vi "Cast Command from Transfer Group.vi"(8 "error in (no error)":errorcluster, 9 "Transfer Group iteration":u64, 10 "Transfer Group id":i32, 11 "Plugin Thread in":refnum<class "Plugin Thread.lvclass">) -> (0 "error out":errorcluster, 2 "command parameters":T1, 3 "Plugin Thread out":refnum<class "Plugin Thread.lvclass">)   [LabVIEW 2021, in "DSF Core.lvlib" / "Plugin Thread.lvclass"]
uses:
  Thread/Plugin/Plugin Thread.lvclass
  Interface/Plugin/Command Parameters.ctl
  Interface/Plugin/Plugin Interface.lvclass
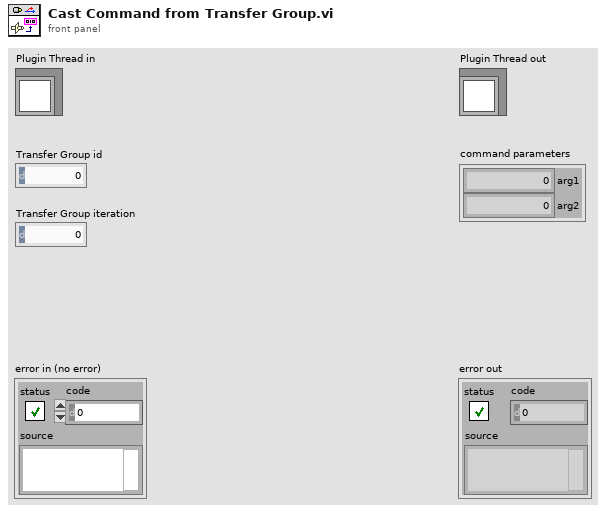
[diagram p1: front panel]
types:
  T1 = typedef "DSF Core.lvlib/Plugin Interface.lvclass/Command Parameters.ctl" = cluster{"arg1":u64, "arg2":u64}
  T2 = cluster{"Transfer Group ID":i32, "unused":i32, "Transfer Group iteration":u64}
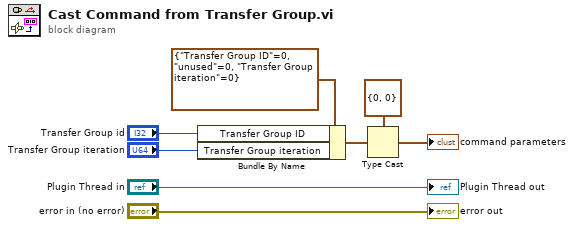
[diagram p0: block diagram]
diagram:
  n1 = Bundle By Name(cluster=T2 {"Transfer Group ID"=0, "unused"=0, "Transfer Group iteration"=0} ("Cluster"), "Transfer Group ID"="Transfer Group id", "Transfer Group iteration"="Transfer Group iteration") -> (w3:T2)
  n2 = Type Cast(type=T1 {"arg1"=0, "arg2"=0} ("command parameters"), x=w3) -> (*(type *) &x=→"command parameters":T1)
  "error out" <- "error in (no error)"
  "Plugin Thread out" <- "Plugin Thread in"
